vi "Flatten to CSV Record (UTF-16).vi"(7 "delimiter (,) *ASCII":string=",\u0000", 10 "error in (no error)":errorcluster, 11 "row of strings *UTF-16":string[](array[string])) -> (2 "error out":errorcluster, 3 "CSV record *UTF-16":string)   [LabVIEW 2013, in "SET_Robust CSV (UTF-16).lvlib"]
doc: "Convert 1D array of ANSI strings into a single CSV record (row).\n\nThe output CSV record string is formatted in accordance with RFC-4180 (see <b>http://tools.ietf.org/html/rfc4180<\\b>). \n\nAll cells containing double quotes (0x22), CR (0x0D) , LF (0x0A) or the delimiter character will be enclosed in double quotes. All double quote characters within a cell will be escaped using a second double quote character. A single LF character is appended to the end of the record.\n\nRev. 0.0 2014-02-20 Ryan Porter\nFirst Draft"
uses:
  SET_Robust CSV (UTF-16).lvlib
panel:
  # "Flatten to CSV Record.vi\n\nConvert 1D array of UTF-16 LE strings into a single CSV record (row). The output CSV record string is formatted in accordance with RFC-4180 (see http://tools.ietf.org/html/rfc4180). \n\nAll cells containing double quotes (0x2200), CR (0x0D00) , LF (0x0A00) or the delimiter character will be enclosed in double quotes. All double quote characters within a cell will be escaped using a second double quote character. A single LF character is appended to the end of the record."
  # "License: BSD (2-Clause) - http://opensource.org/licenses/BSD-2-Clause \n\nCopyright (c) 2014, Ryan Porter\nAll rights reserved."
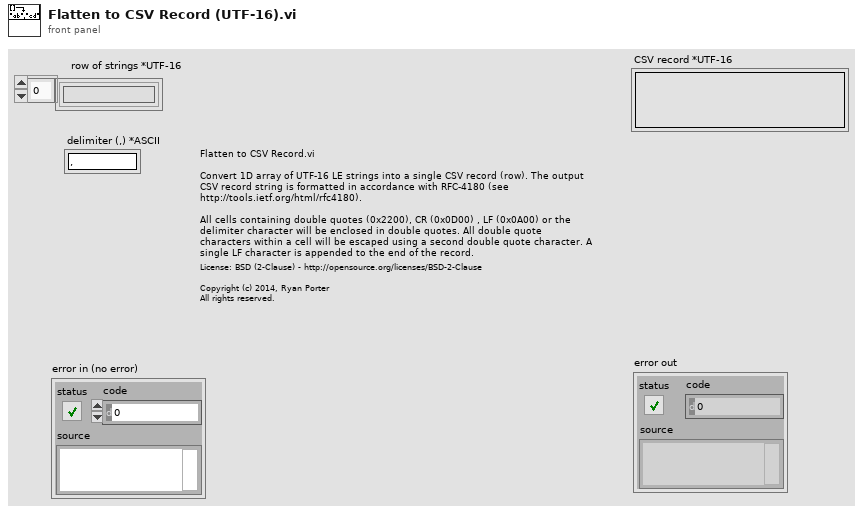
[diagram p1: front panel]
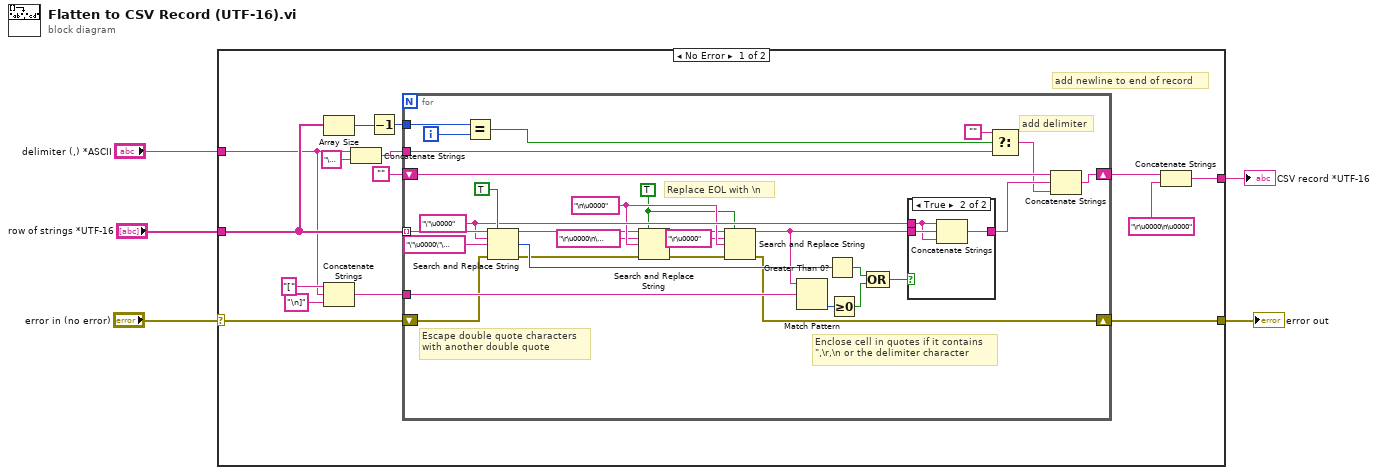
[diagram p0: block diagram]
diagram:
  n1 = case shown="No Error" "error in (no error)" {
    selector: "error in (no error)" -> [w10 w55]
    tunnel: "row of strings *UTF-16" -> [w18 _]
    tunnel: "delimiter (,) *ASCII" -> [w7 _]
    tunnel: [w11 _] -> w3
    tunnel: [w9 w55] -> w1
    frame No Error {
      # "add newline to end of record"
      n2 = Array Size(array=w18) -> (size(s)=w17:i32)
      n3 = Concatenate Strings("[", w7, "\n]") -> (w14:string)
      n4 = Concatenate Strings(w7, "\u0000" ("string")) -> (w8:string)
      n5 = Decrement(x=w17) -> (x-1=w19:i32)
      n6 = for {
        tunnel: w18 -> [w50] mode=indexing
        tunnel: w14 -> [w42]
        shift-right: [w46] -> w13
        shift-left: "" -> [w45]
        tunnel: w8 -> [w39]
        tunnel: w19 -> [w36]
        shift-right: [w21] -> w9
        shift-left: w10 -> [w31]
        i -> [w41]
        w27 = TRUE ("replace all? (F)")
        w30 = "\n\u0000" ("search string")
        w47 = "\"\u0000" ("search string")
        # "Replace EOL with \\n"
        # "Escape double quote characters\nwith another double quote"
        # "Enclose cell in quotes if it contains\n\",\\r,\\n or the delimiter character"
        # "add delimiter"
        n7 = Equal?(x=w36, y=w41) -> (x = y?=w40:bool)
        n8 = Search and Replace String(replace all?=TRUE ("replace all? (F)"), input string=w50, search string=w47, replace string="\"\u0000\"\u0000" ("replace string (\"\")"), error in=w31) -> (result string=w24:string, number of replacements=w35:i32, error out=w22:errorcluster)  [unwired: 3 in, 1 out]
        n9 = Search and Replace String(replace all?=w27, input string=w24, search string="\r\u0000\n\u0000", replace string=w30, error in=w22) -> (result string=w25:string, error out=w29:errorcluster)  [unwired: 3 in, 2 out]
        n10 = Search and Replace String(replace all?=w27, input string=w25, search string="\r\u0000", replace string=w30, error in=w29) -> (result string=w23:string, error out=w21:errorcluster)  [unwired: 3 in, 2 out]
        n11 = Match Pattern(string=w23, regular expression=w42) -> (offset past match=w43:i32)  [unwired: 1 in, 3 out]
        n12 = Greater Than 0?(x=w35) -> (x > 0?=w34:bool)
        n13 = Greater Or Equal To 0?(x=w43) -> (x >= 0?=w33:bool)
        n14 = Compound Arithmetic op=OR(w34, w33) -> (w32:bool)
        n15 = case shown="True" w32 {
          tunnel: w23 -> [w51 w54]
          tunnel: w47 -> [_ w53]
          tunnel: [w51 w52] -> w44
          frame False {
          }
          frame True {
            n16 = Concatenate Strings(w53, w54, w53) -> (w52:string)
          }
        }
        n17 = Select(t="", s=w40, f=w39) -> (s? t:f=w37:string)
        n18 = Concatenate Strings(w45, w44, w37) -> (w46:string)
      }
      n19 = Concatenate Strings(w13, "\r\u0000\n\u0000") -> (w11:string)
    }
    frame Error {
    }
  }
  "CSV record *UTF-16" <- w3
  "error out" <- w1
